vi "RydbergExpControl_2014.09.11_beta.vi"() -> ()   [LabVIEW 2013]
uses:
  AndorCamera/camera_controls.ctl
  <userlib>/atmcd32d.llb/AcquisitionMode_mode typedef.ctl
  <userlib>/atmcd32d.llb/TriggerMode_mode typedef.ctl
  6704/6704_static_voltages_control.ctl
  rydberg_state_machine_states.ctl
panel:
  out "Waveform Chart":dbl(graph)
  in  "Count Number?":bool
  out "Number":dbl format="%^#_6g"
  out "OD":dbl[][](graph)
  out "Atom Closeup":dbl[][](graph)
  out "Atoms - BG":dbl[][](graph)
  out "error out":errorcluster
  out "error constant":errorcluster
  out "Array":dbl[](array[numeric])
  out "Background Image":i16[][](graph)
  out "Atom Image":i16[][](graph)
  in  "Tab Control":T1(tab)
  in  "Trigger Snap Mode":bool
  out "Camera Ready":bool
  in  "Scan Name":string
  in  "Raw_Data Folder":path
  out "Exp Running":bool
  in  "PB Instruction Time To Change":i32
  in  "Static Channel To Change":i32
  in  "Step Size":dbl min=1e-06
  in  "Final Value":dbl
  in  "Initial Value":dbl
  out "You Are Changing:":string
  in  "Shutdown Experiment":bool
  in  "Start Experiment":bool
  in  "Instructions":T2(array[cluster])=[{"Instruct Data"=0, "Op Code"=0, "Flags"=[TRUE, FALSE, FALSE, FALSE, FALSE, FALSE, FALSE, FALSE, FALSE, FALSE, FALSE, FALSE, FALSE, FALSE, FALSE, FALSE, FALSE, FALSE, FALSE, FALSE, FALSE, FALSE, FALSE, FALSE], "Comments"="", "Time (s)"=0.1}, {"Instruct Data"=0, "Op Code"=0, "Flags"=[FALSE, FALSE, FALSE, FALSE, FALSE, FALSE, FALSE, FALSE, FALSE, FALSE, FALSE, FALSE, FALSE, FALSE, FALSE, FALSE, FALSE, FALSE, FALSE, FALSE, FALSE, FALSE, FALSE, FALSE], "Comments"="", "Time (s)"=0.1}, {"Instruct Data"=0, "Op Code"=0, "Flags"=[TRUE, FALSE, FALSE, FALSE, FALSE, FALSE, FALSE, FALSE, FALSE, FALSE, FALSE, FALSE, FALSE, FALSE, FALSE, FALSE, FALSE, FALSE, FALSE, FALSE, FALSE, FALSE, FALSE, FALSE], "Comments"="", "Time (s)"=0.1}, {"Instruct Data"=0, "Op Code"=6, "Flags"=[FALSE, FALSE, FALSE, FALSE, FALSE, FALSE, FALSE, FALSE, FALSE, FALSE, FALSE, FALSE, FALSE, FALSE, FALSE, FALSE, FALSE, FALSE, FALSE, FALSE, FALSE, FALSE, FALSE, FALSE], "Comments"="", "Time (s)"=0.1}] {"Time (s)" format="%.3p"; "Op Code" items=["Continue", "Stop", "Loop", "End Loop", "JSR", "RTS", "Branch", "Long Delay", "Wait"]}
  in  "What To Change":enum16{"PulseBlaster", "Static Voltage"}(ring)=enum."Static Voltage"
  out "Scan Progress":dbl(slide) caption="Slide" scale=0.0..100.0
  out "Camera Information":T3 {"VS Speed (us)" format="%.2f"}
  in  "Acquisition Parameters":T4={"Acquisition Mode"=enum."Kinetics", "Trigger Mode"=enum."External", "Frame \nTransfer"=FALSE, "Exposure Time (s)"=0.0001, "Accumulation Cycle Time (s)"=0.0, "# Accumulations"=1, "# Kinetics"=2, "Kinetic Cycle Time (s)"=0.0, "Horizontal Bin Size"=1, "Vertical Bin Size"=1} {"Vertical Bin Size" min=1; "Horizontal Bin Size" min=1; "Kinetic Cycle Time (s)" format="%.2f"; "# Kinetics" min=1; "# Accumulations" min=1; "Accumulation Cycle Time (s)" format="%.2f"; "Exposure Time (s)" format="%.2e"}
  out "Calcualted Times":T7 {"Kinetic" format="%.4f"; "Accumulate" format="%.4f"; "Exposure" format="%.4f"}
  in  "Red MOT 87 Inputs":T8={"Active Device"="6733_Red_87", "Active Channels"=[TRUE, FALSE, FALSE, FALSE, FALSE, FALSE, FALSE, FALSE], "Waveform Parameters"=[[{"Functional Form"=enum."Polynomial", "Start Voltage"=0.0, "End Voltage"=0.0, "Time"=0.0, "Degree"=1, "Sample Rate"=0.0}, {"Functional Form"=enum."Exponential", "Start Voltage"=0.0, "End Voltage"=0.0, "Time"=0.0, "Degree"=1, "Sample Rate"=0.0}, {"Functional Form"=enum."Exponential", "Start Voltage"=0.0, "End Voltage"=0.0, "Time"=0.0, "Degree"=1, "Sample Rate"=0.0}, {"Functional Form"=enum."Exponential", "Start Voltage"=0.0, "End Voltage"=0.0, "Time"=0.0, "Degree"=1, "Sample Rate"=0.0}, {"Functional Form"=enum."Exponential", "Start Voltage"=0.0, "End Voltage"=0.0, "Time"=0.0, "Degree"=1, "Sample Rate"=0.0}, {"Functional Form"=enum."Exponential", "Start Voltage"=0.0, "End Voltage"=0.0, "Time"=0.0, "Degree"=1, "Sample Rate"=0.0}], [{"Functional Form"=enum."Exponential", "Start Voltage"=0.0, "End Voltage"=0.0, "Time"=0.0, "Degree"=1, "Sample Rate"=0.0}, {"Functional Form"=enum."Exponential", "Start Voltage"=0.0, "End Voltage"=0.0, "Time"=0.0, "Degree"=1, "Sample Rate"=0.0}, {"Functional Form"=enum."Exponential", "Start Voltage"=0.0, "End Voltage"=0.0, "Time"=0.0, "Degree"=1, "Sample Rate"=0.0}, {"Functional Form"=enum."Exponential", "Start Voltage"=0.0, "End Voltage"=0.0, "Time"=0.0, "Degree"=1, "Sample Rate"=0.0}, {"Functional Form"=enum."Exponential", "Start Voltage"=0.0, "End Voltage"=0.0, "Time"=0.0, "Degree"=1, "Sample Rate"=0.0}, {"Functional Form"=enum."Exponential", "Start Voltage"=0.0, "End Voltage"=0.0, "Time"=0.0, "Degree"=1, "Sample Rate"=0.0}], [{"Functional Form"=enum."Exponential", "Start Voltage"=0.0, "End Voltage"=0.0, "Time"=0.0, "Degree"=1, "Sample Rate"=0.0}, {"Functional Form"=enum."Exponential", "Start Voltage"=0.0, "End Voltage"=0.0, "Time"=0.0, "Degree"=1, "Sample Rate"=0.0}, {"Functional Form"=enum."Exponential", "Start Voltage"=0.0, "End Voltage"=0.0, "Time"=0.0, "Degree"=1, "Sample Rate"=0.0}, {"Functional Form"=enum."Exponential", "Start Voltage"=0.0, "End Voltage"=0.0, "Time"=0.0, "Degree"=1, "Sample Rate"=0.0}, {"Functional Form"=enum."Exponential", "Start Voltage"=0.0, "End Voltage"=0.0, "Time"=0.0, "Degree"=1, "Sample Rate"=0.0}, {"Functional Form"=enum."Exponential", "Start Voltage"=0.0, "End Voltage"=0.0, "Time"=0.0, "Degree"=1, "Sample Rate"=0.0}], [{"Functional Form"=enum."Exponential", "Start Voltage"=0.0, "End Voltage"=0.0, "Time"=0.0, "Degree"=1, "Sample Rate"=0.0}, {"Functional Form"=enum."Exponential", "Start Voltage"=0.0, "End Voltage"=0.0, "Time"=0.0, "Degree"=1, "Sample Rate"=0.0}, {"Functional Form"=enum."Exponential", "Start Voltage"=0.0, "End Voltage"=0.0, "Time"=0.0, "Degree"=1, "Sample Rate"=0.0}, {"Functional Form"=enum."Exponential", "Start Voltage"=0.0, "End Voltage"=0.0, "Time"=0.0, "Degree"=1, "Sample Rate"=0.0}, {"Functional Form"=enum."Exponential", "Start Voltage"=0.0, "End Voltage"=0.0, "Time"=0.0, "Degree"=1, "Sample Rate"=0.0}, {"Functional Form"=enum."Exponential", "Start Voltage"=0.0, "End Voltage"=0.0, "Time"=0.0, "Degree"=1, "Sample Rate"=0.0}], [{"Functional Form"=enum."Exponential", "Start Voltage"=0.0, "End Voltage"=0.0, "Time"=0.0, "Degree"=1, "Sample Rate"=0.0}, {"Functional Form"=enum."Exponential", "Start Voltage"=0.0, "End Voltage"=0.0, "Time"=0.0, "Degree"=1, "Sample Rate"=0.0}, {"Functional Form"=enum."Exponential", "Start Voltage"=0.0, "End Voltage"=0.0, "Time"=0.0, "Degree"=1, "Sample Rate"=0.0}, {"Functional Form"=enum."Exponential", "Start Voltage"=0.0, "End Voltage"=0.0, "Time"=0.0, "Degree"=1, "Sample Rate"=0.0}, {"Functional Form"=enum."Exponential", "Start Voltage"=0.0, "End Voltage"=0.0, "Time"=0.0, "Degree"=1, "Sample Rate"=0.0}, {"Functional Form"=enum."Exponential", "Start Voltage"=0.0, "End Voltage"=0.0, "Time"=0.0, "Degree"=1, "Sample Rate"=0.0}], [{"Functional Form"=enum."Exponential", "Start Voltage"=0.0, "End Voltage"=0.0, "Time"=0.0, "Degree"=1, "Sample Rate"=0.0}, {"Functional Form"=enum."Exponential", "Start Voltage"=0.0, "End Voltage"=0.0, "Time"=0.0, "Degree"=1, "Sample Rate"=0.0}, {"Functional Form"=enum."Exponential", "Start Voltage"=0.0, "End Voltage"=0.0, "Time"=0.0, "Degree"=1, "Sample Rate"=0.0}, {"Functional Form"=enum."Exponential", "Start Voltage"=0.0, "End Voltage"=0.0, "Time"=0.0, "Degree"=1, "Sample Rate"=0.0}, {"Functional Form"=enum."Exponential", "Start Voltage"=0.0, "End Voltage"=0.0, "Time"=0.0, "Degree"=1, "Sample Rate"=0.0}, {"Functional Form"=enum."Exponential", "Start Voltage"=0.0, "End Voltage"=0.0, "Time"=0.0, "Degree"=1, "Sample Rate"=0.0}], [{"Functional Form"=enum."Exponential", "Start Voltage"=0.0, "End Voltage"=0.0, "Time"=0.0, "Degree"=1, "Sample Rate"=0.0}, {"Functional Form"=enum."Exponential", "Start Voltage"=0.0, "End Voltage"=0.0, "Time"=0.0, "Degree"=1, "Sample Rate"=0.0}, {"Functional Form"=enum."Exponential", "Start Voltage"=0.0, "End Voltage"=0.0, "Time"=0.0, "Degree"=1, "Sample Rate"=0.0}, {"Functional Form"=enum."Exponential", "Start Voltage"=0.0, "End Voltage"=0.0, "Time"=0.0, "Degree"=1, "Sample Rate"=0.0}, {"Functional Form"=enum."Exponential", "Start Voltage"=0.0, "End Voltage"=0.0, "Time"=0.0, "Degree"=1, "Sample Rate"=0.0}, {"Functional Form"=enum."Exponential", "Start Voltage"=0.0, "End Voltage"=0.0, "Time"=0.0, "Degree"=1, "Sample Rate"=0.0}], [{"Functional Form"=enum."Exponential", "Start Voltage"=0.0, "End Voltage"=0.0, "Time"=0.0, "Degree"=1, "Sample Rate"=0.0}, {"Functional Form"=enum."Exponential", "Start Voltage"=0.0, "End Voltage"=0.0, "Time"=0.0, "Degree"=1, "Sample Rate"=0.0}, {"Functional Form"=enum."Exponential", "Start Voltage"=0.0, "End Voltage"=0.0, "Time"=0.0, "Degree"=1, "Sample Rate"=0.0}, {"Functional Form"=enum."Exponential", "Start Voltage"=0.0, "End Voltage"=0.0, "Time"=0.0, "Degree"=1, "Sample Rate"=0.0}, {"Functional Form"=enum."Exponential", "Start Voltage"=0.0, "End Voltage"=0.0, "Time"=0.0, "Degree"=1, "Sample Rate"=0.0}, {"Functional Form"=enum."Exponential", "Start Voltage"=0.0, "End Voltage"=0.0, "Time"=0.0, "Degree"=1, "Sample Rate"=1.0}]], "Active Phases"=[TRUE, FALSE, FALSE, FALSE, FALSE, FALSE], "Phase Times"=[0.001], "Trigger Channel"="/6733_Red_87/PFI0"} {"Phase Times" format="%.0p"; "Waveform Parameters"."Degree" min=1}
  in  "6704 Static Voltage Settings":T9={"Device Name"="6704_Static", "Voltages"=[5.0, 0.0, 0.0, 0.0, 0.0, 0.0, 0.0, 0.0, 0.0, 0.0, 0.0, 0.0, 0.0, 0.0, 0.0, 0.0]}
  out "Andor Initialization Error Codes":T10
  out "Acq. Error Codes":T11
  out "Tree":string(tree)
  # "(1) 461 MOT beams"
  # "(2) Imaging AOM 1"
  # "(3) Imaging AOM 2"
  # "(4) Camera"
  # "(5) Zeeman shutter"
  # "(6) Repumper shutter"
  # "(7) 461 MOT coils"
  # "(8) 689 MOT coils"
  # "(9) 87 Sr Red MOT Trig"
  # "(10) ??? Shutter"
  # "(11) Red AOM"
  # "(12) Sat Abs Current Switch"
  # "(13) Zeeman MOSFET"
  # "1"
  # "2"
  # "3"
  # "4"
  # "5"
  # "6"
  # "7"
  # "8"
  # "9"
  # "10"
  # "11"
  # "12"
  # "13"
  # "14"
  # "15"
  # "16"
  # "17"
  # "18"
  # "19"
  # "20"
  # "21"
  # "22"
  # "23"
  # "24"
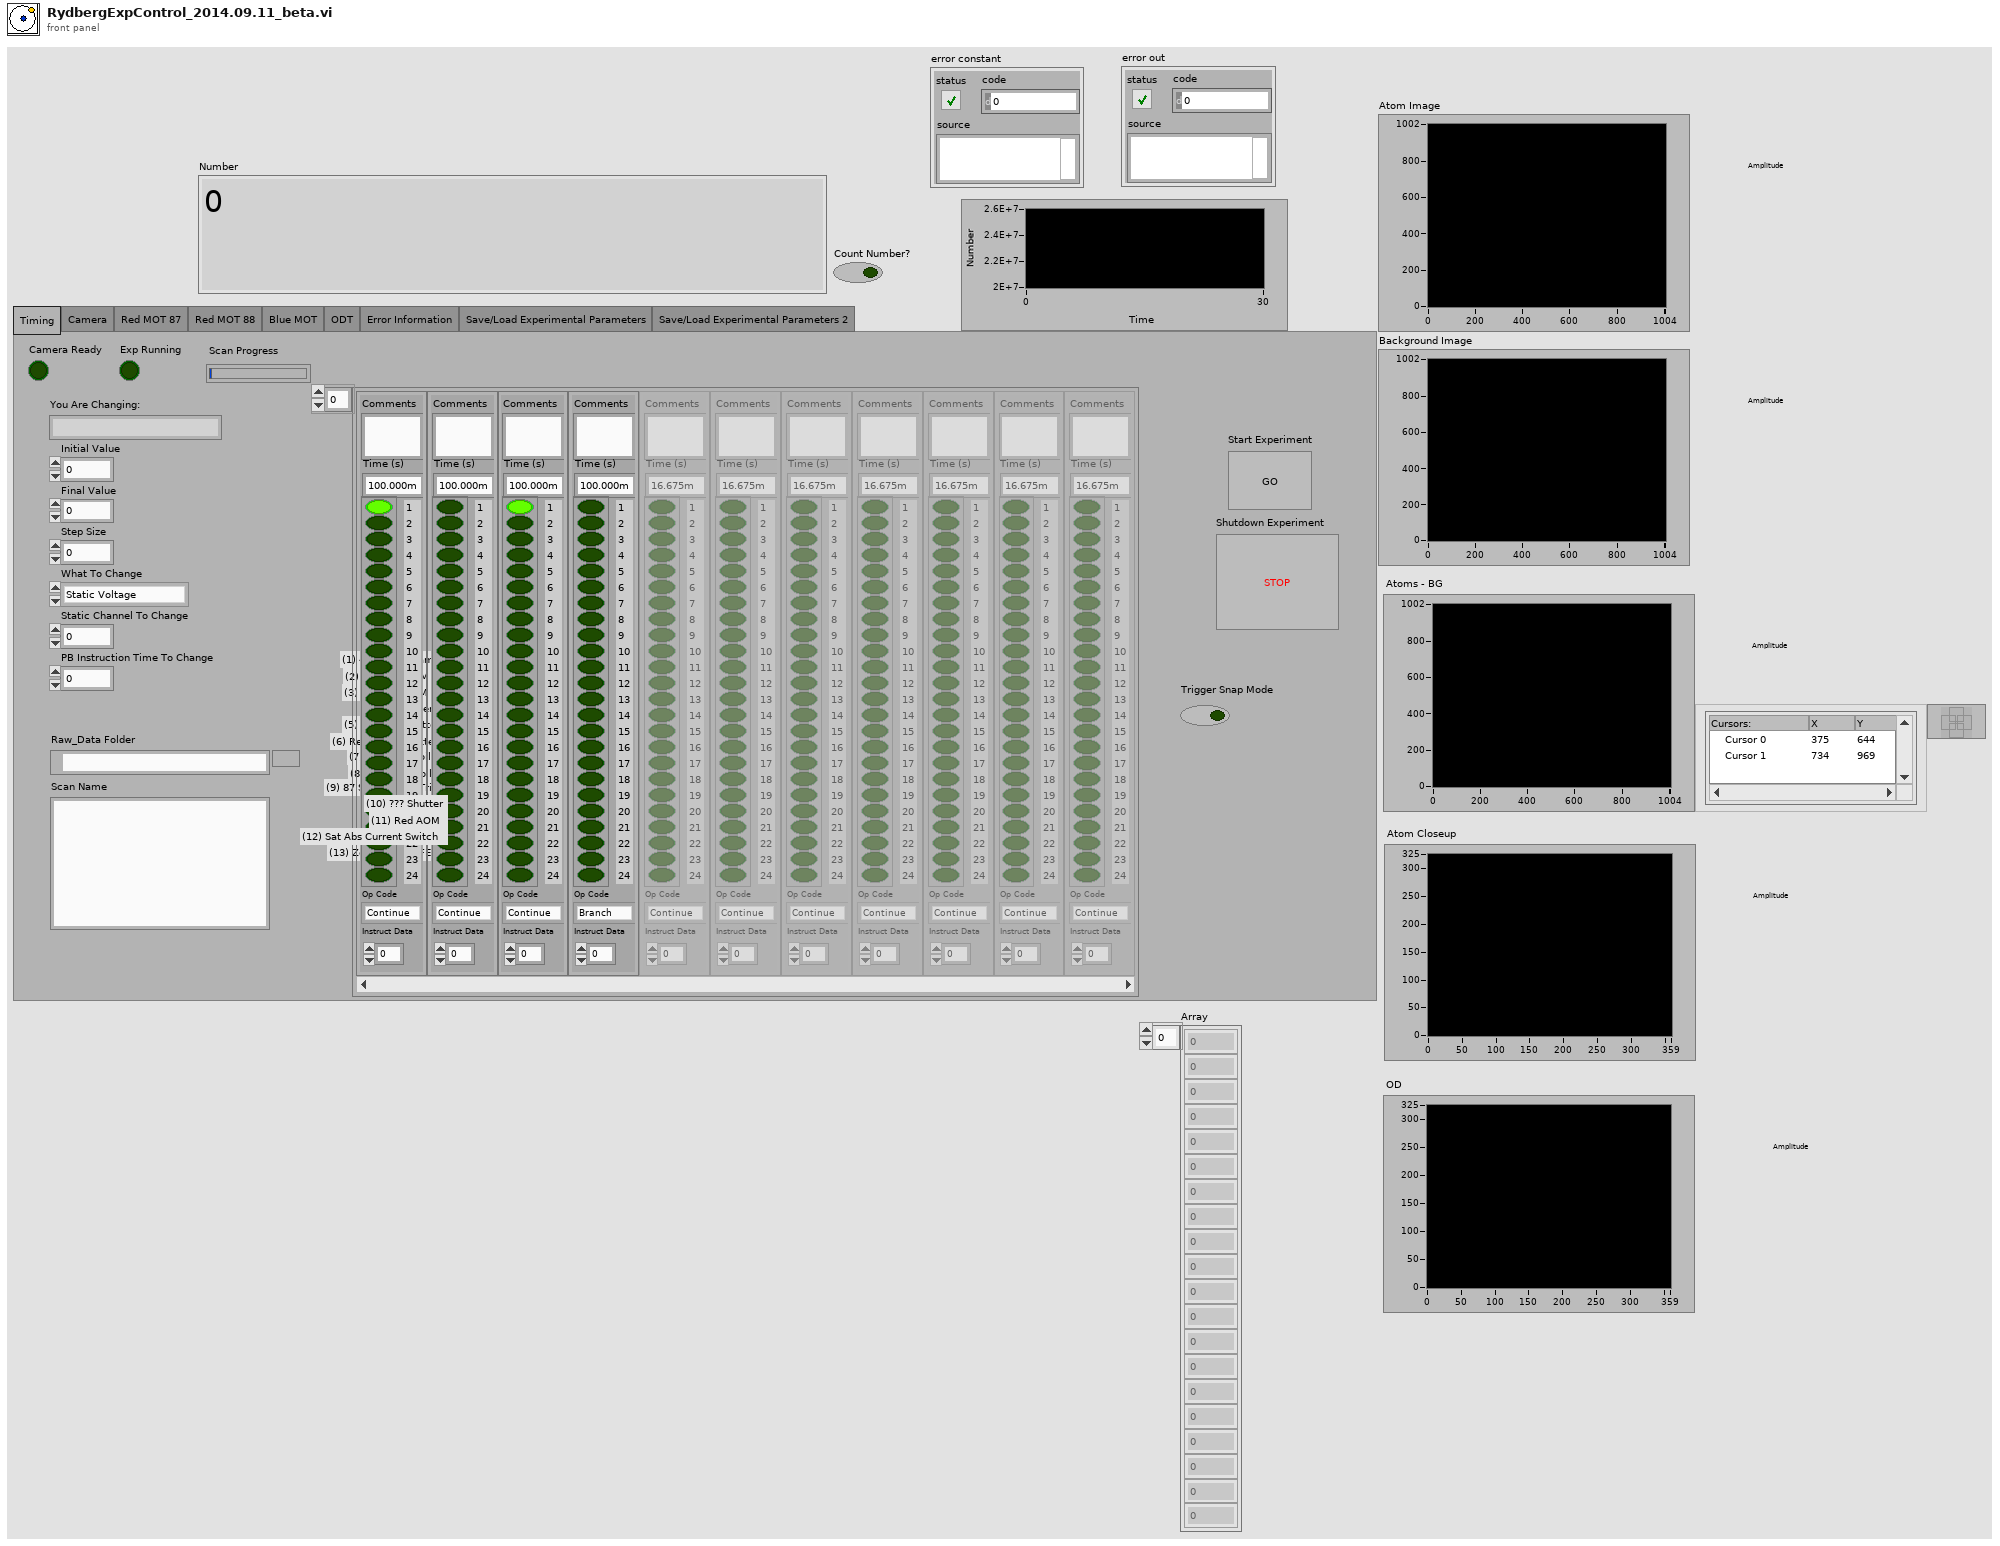
[diagram p1: front panel]
types:
  T1 = enum32{"Timing", "Camera", "Red MOT 87", "Red MOT 88", "Blue MOT", "ODT", "Error Information", "Save/Load Experimental Parameters", "Save/Load Experimental Parameters 2"}
  T2 = cluster{"Instruct Data":i32, "Op Code":i32, "Flags":bool[], "Comments":string, "Time (s)":dbl}[]
  T3 = cluster{"xpixels":i32, "ypixels":i32, "# VS Speeds":i32, "VS Speed (us)":sgl, "Temperature Stable":bool, "Temperature (C)":i32}
  T4 = typedef "camera_controls.ctl" = cluster{"Acquisition Mode":T5, "Trigger Mode":T6, "Frame \nTransfer":bool, "Exposure Time (s)":sgl, "Accumulation Cycle Time (s)":sgl, "# Accumulations":i32, "# Kinetics":i32, "Kinetic Cycle Time (s)":sgl, "Horizontal Bin Size":i32, "Vertical Bin Size":i32}
  T5 = typedef "AcquisitionMode_mode typedef.ctl" = enum16{"Reserved (0)", "Single Scan", "Accumulate", "Kinetics", "Fast Kinetics", "Run Till Abort", "Reserved (6)", "Reserved (7)", "Reserved (8)", "Time Delayed Integration"}
  T6 = typedef "TriggerMode_mode typedef.ctl" = enum16{"Internal", "External", "N/A (2)", "N/A (3)", "N/A (4)", "N/A (5)", "External Start", "External Exposure (Bulb)", "N/A (8)", "External FVB EM", "Software", "N/A (11)", "External Charge Shifting"}
  T7 = cluster{"Exposure":sgl, "Accumulate":sgl, "Kinetic":sgl}
  T8 = cluster{"Active Device":string, "Active Channels":bool[], "Waveform Parameters":cluster{"Functional Form":enum16{"Polynomial", "Exponential"}, "Start Voltage":dbl, "End Voltage":dbl, "Time":dbl, "Degree":i8, "Sample Rate":dbl}[][], "Active Phases":bool[], "Phase Times":dbl[], "Trigger Channel":tag}
  T9 = typedef "6704_static_voltages_control.ctl" = cluster{"Device Name":string, "Voltages":dbl[]}
  T10 = cluster{"Initalize Error Code":u32, "GetDetector Error Code":u32, "Get#VSSpeeds Error Code":u32, "Set VS Speed Error":u32, "CoolerOn Error Code":u32, "GetTemperature Error Code":u32, "Shutdown Error Code":u32}
  T11 = cluster{"Set Acq. Mode Error":u32, "Set Trigger Mode Error":u32, "Set FT Error Code":u32, "Set Exposure Time Error Code":u32, "Set Accum Time Error":u32, "Set # Accum Error":u32, "Set # Kinetics Error":u32, "SetKinCycleTime Error":u32}
  T12 = typedef "rydberg_state_machine_states.ctl" = enum16{"Initialize", "Idle", "Trigger Snap Mode", "Scan Mode", "Load Experiment", "Shutdown"}
  T13 = cluster{"6704 Static Voltage Settings":T9, "Instructions":cluster{"Instruct Data":i32, "Op Code":i32, "Flags":bool[], "Comments":string, "Time (s)":dbl}[], "Red MOT 87 Inputs":cluster{"Active Device":string, "Active Channels":bool[], "Waveform Parameters":cluster{"Functional Form":enum16{"Polynomial", "Exponential"}, "Start Voltage":dbl, "End Voltage":dbl, "Time":dbl, "Degree":i8, "Sample Rate":dbl}[][], "Active Phases":bool[], "Phase Times":dbl[], "Trigger Channel":tag}}
  T14 = typedef "LVCursorListTypeDef.ctl" = cluster{"Name":string, "Color":u32, "Style":u8, "Point Style":u8, "Name Visible":bool, "Allow Drag":bool, "Cursor Mode":u32, "Plot":i32, "Index":i32, "Position":cluster{"X":dbl, "Y":dbl}, "X Scale":u32, "Y Scale":u32, "Watch Plots":i32[], "Watch All Plots":bool, "Plot Area":i32, "Label Offset":cluster{"X":dbl, "Y":dbl}}[]
  T15 = cluster{"Instruct Data":i32, "Op Code":i32, "Flags":bool[], "Comments":string, "Time (s)":dbl}
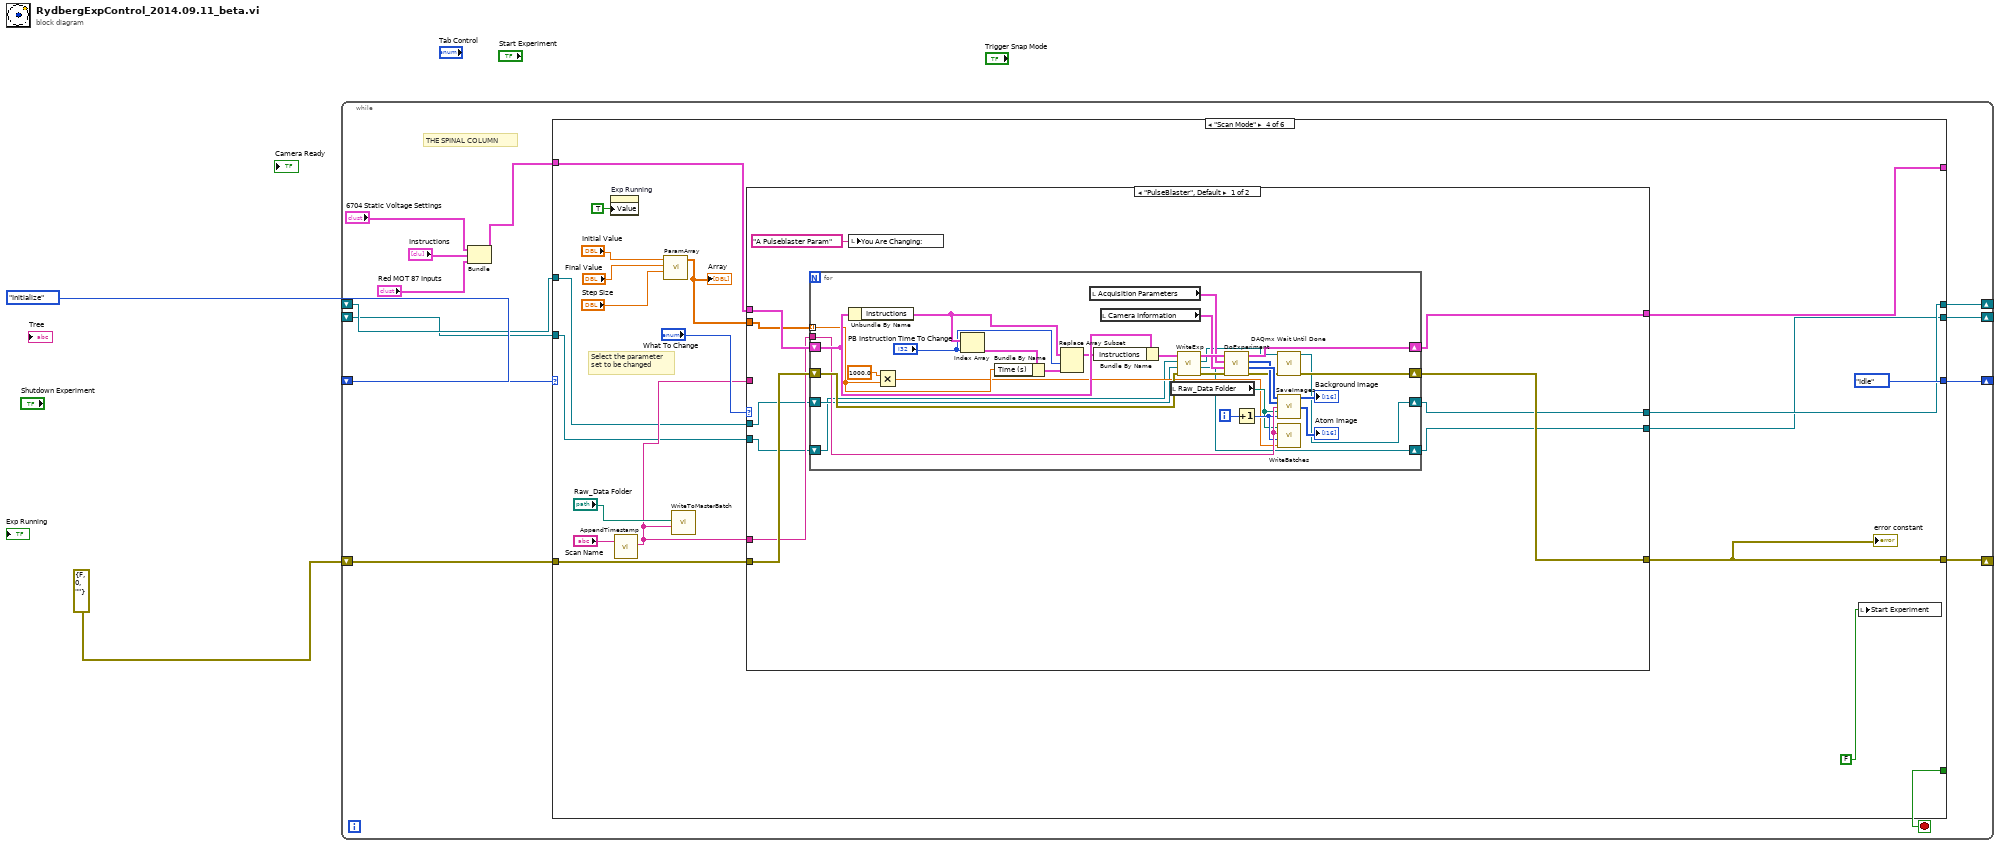
[diagram p0: block diagram]
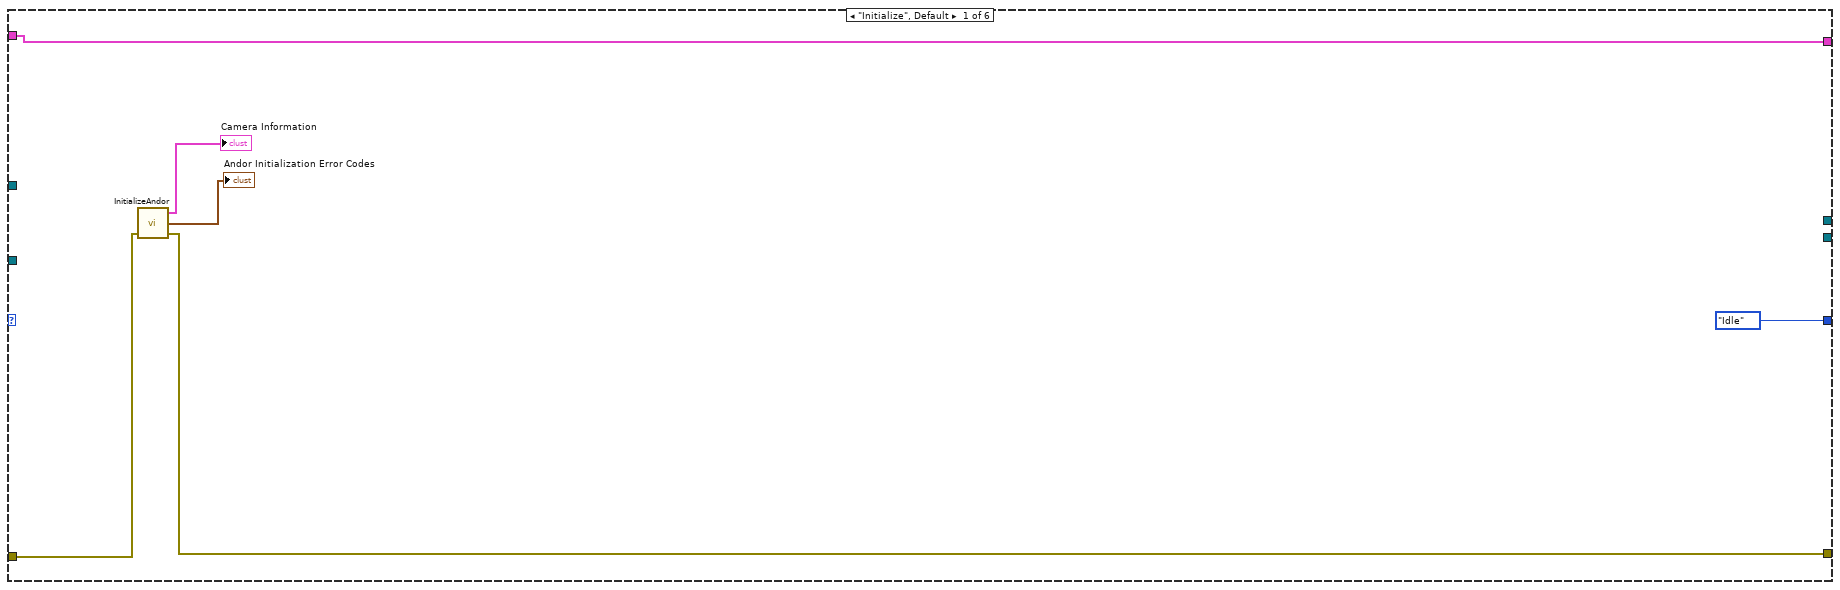
[diagram p2: hidden frame]
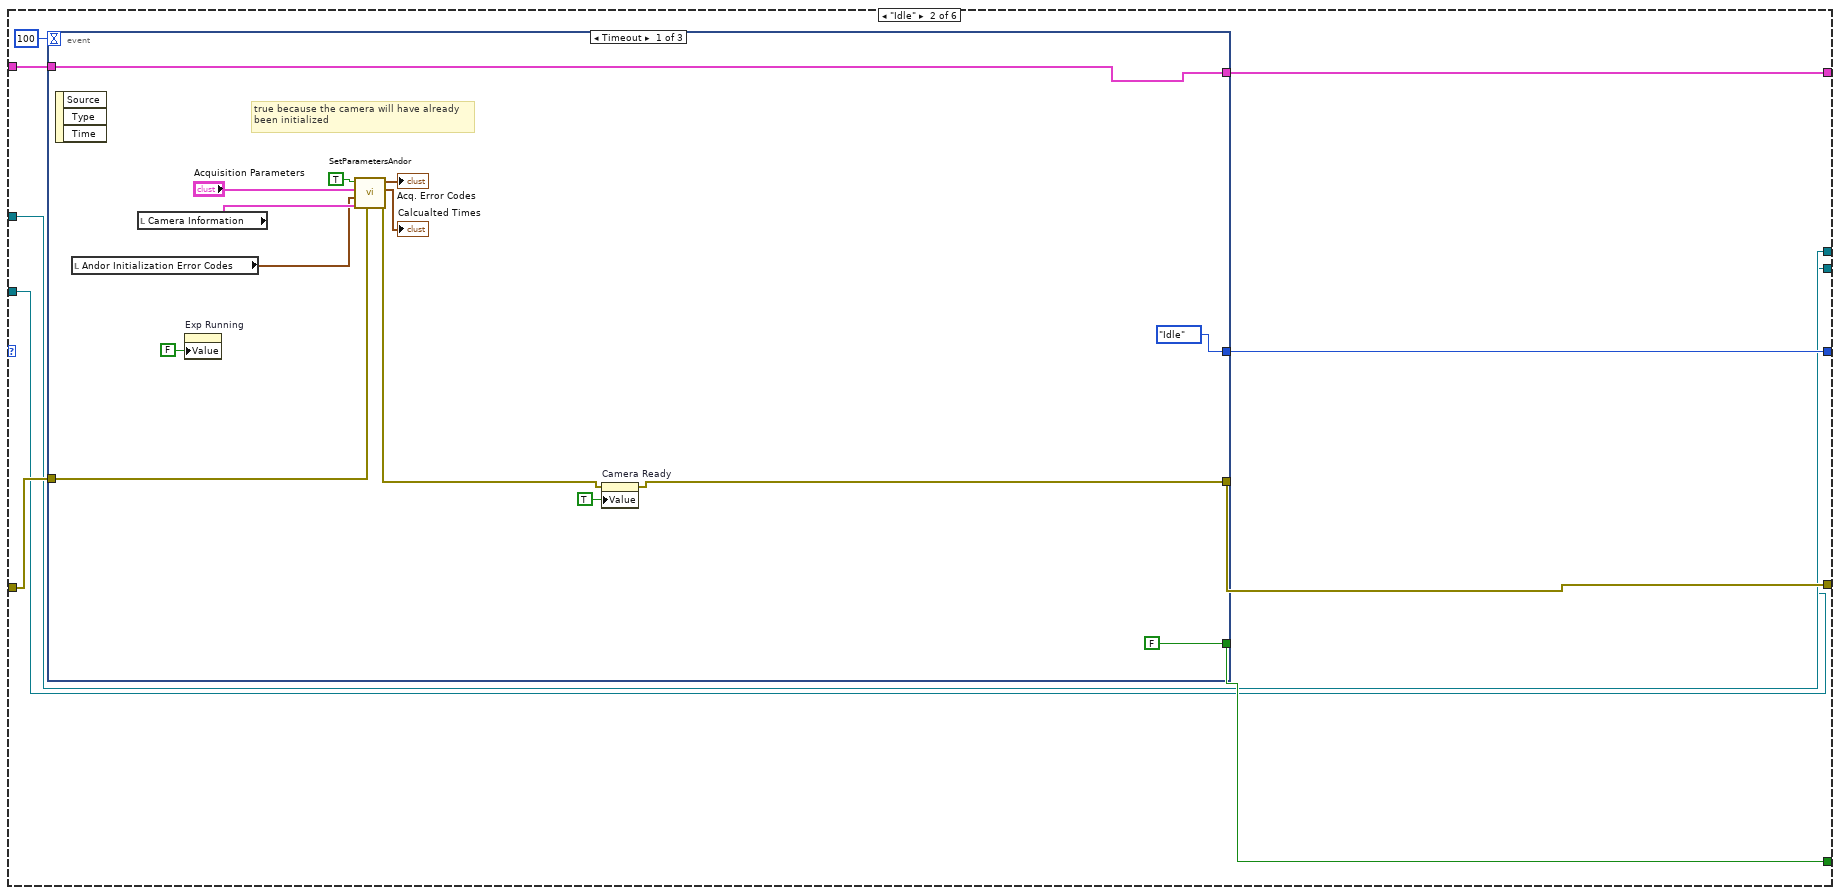
[diagram p3: hidden frame]
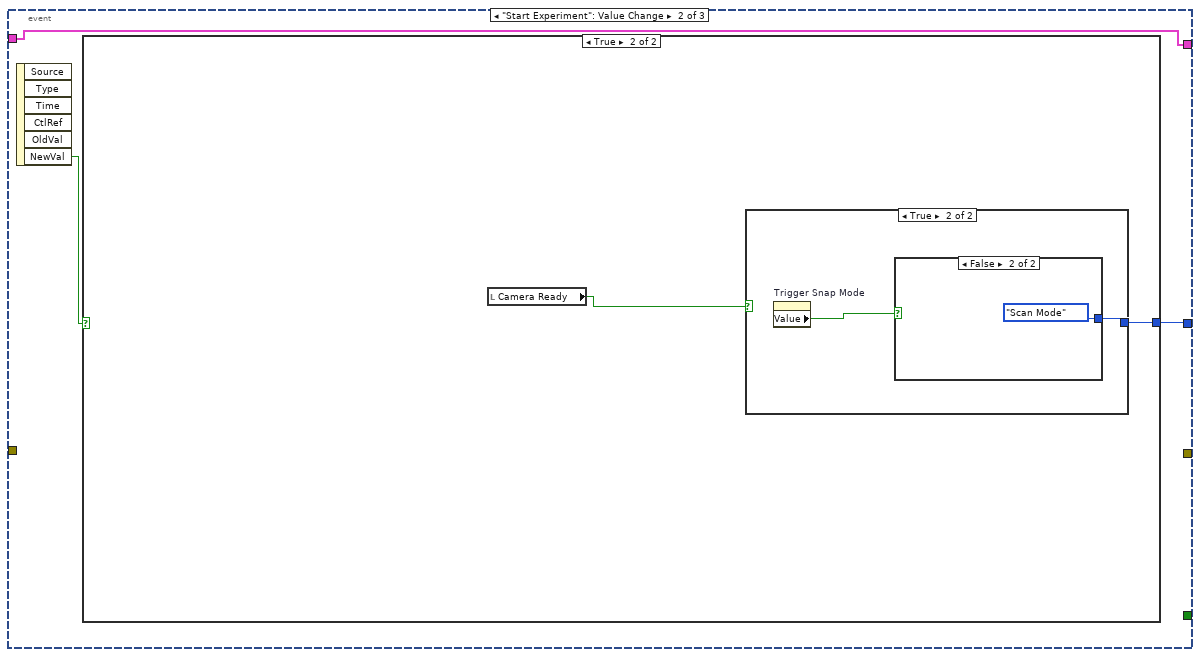
[diagram p4: hidden frame]
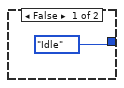
[diagram p5: hidden frame]
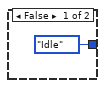
[diagram p6: hidden frame]
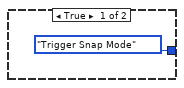
[diagram p7: hidden frame]
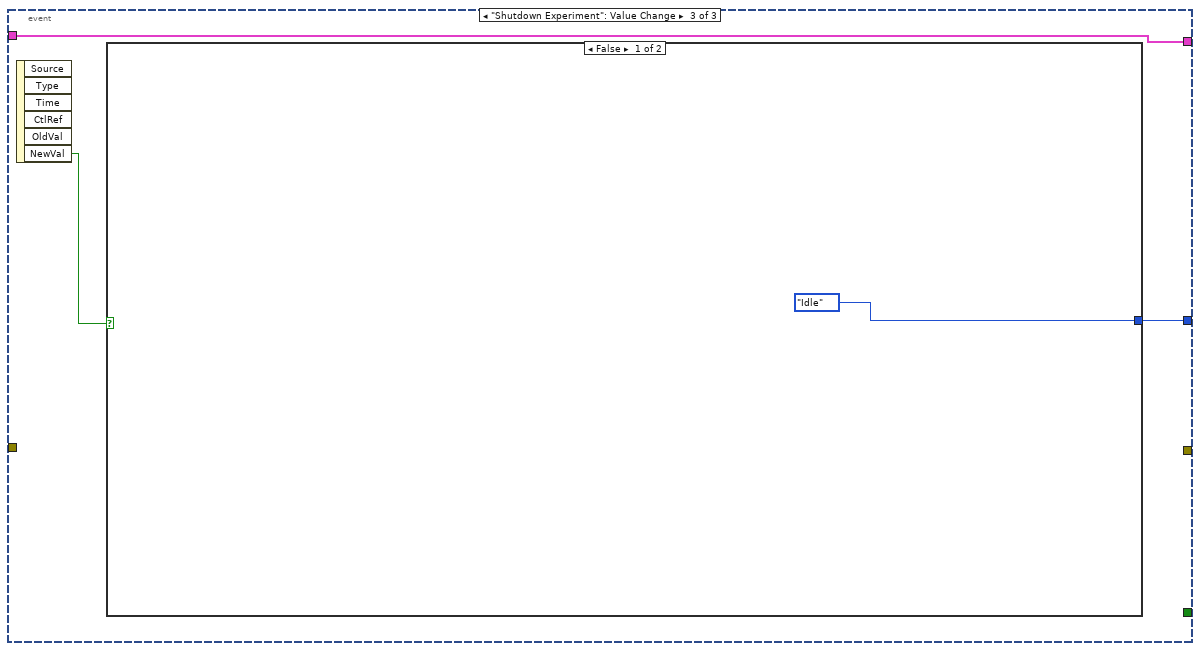
[diagram p8: hidden frame]
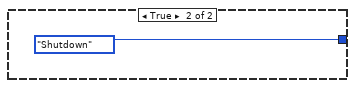
[diagram p9: hidden frame]
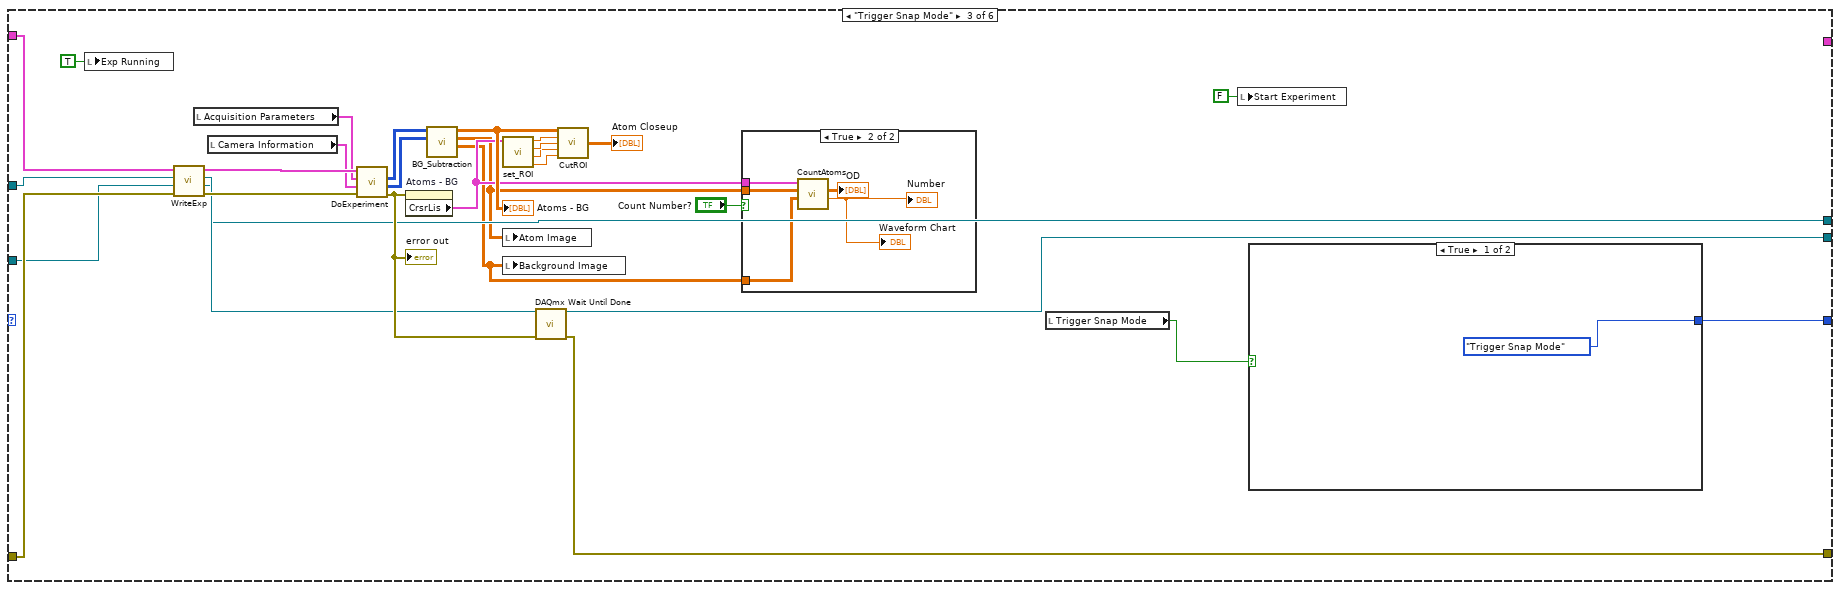
[diagram p10: hidden frame]
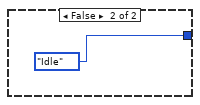
[diagram p12: hidden frame]
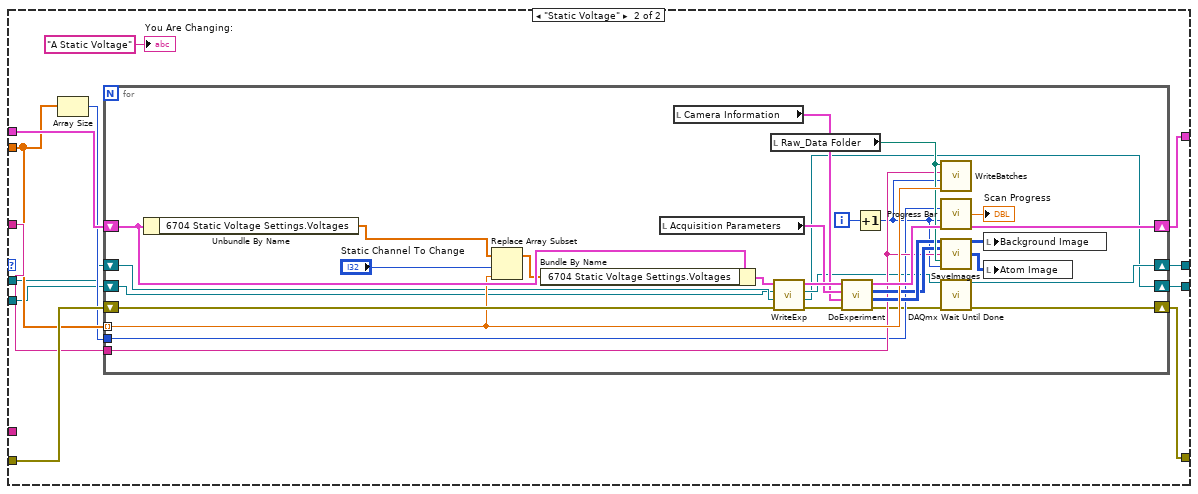
[diagram p13: hidden frame]
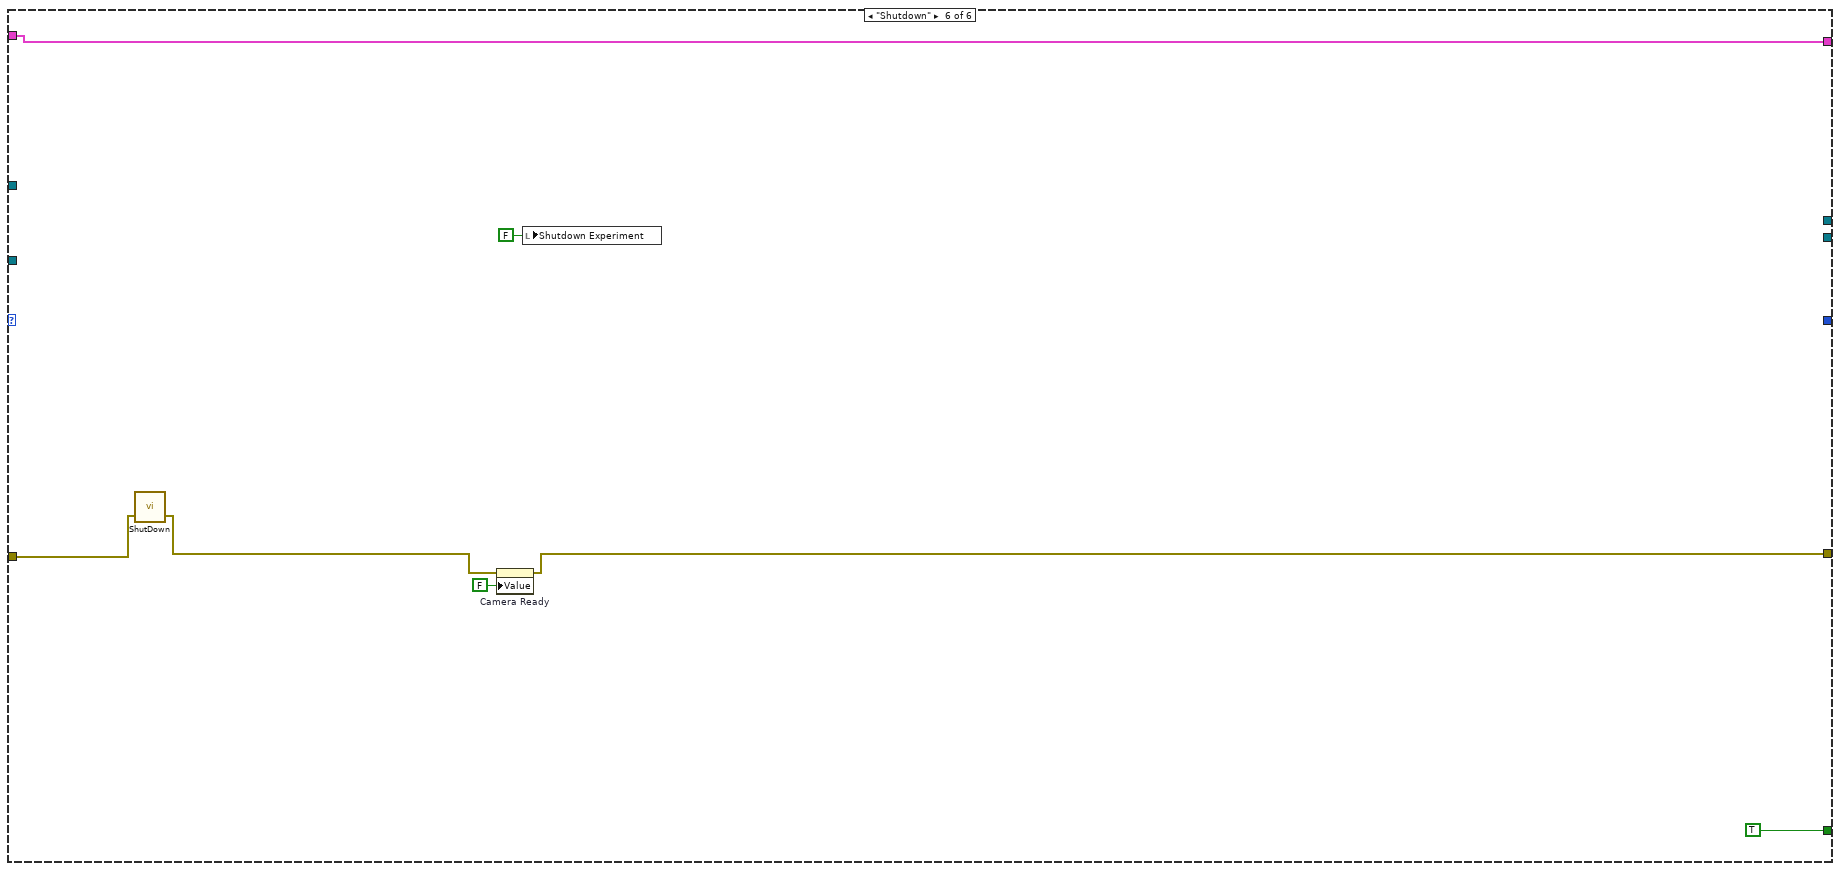
[diagram p15: hidden frame]
diagram:
  n1 = while {
    shift-right: [w12] -> _
    shift-left: rydberg_state_machine_states."Initialize" -> [w15]
    shift-right: [w13] -> _
    shift-left: errorcluster {"status"=FALSE, "code"=0, "source"=""} ("error constant") -> [w14]
    shift-right: [w6] -> _
    shift-left: _ -> [w5]
    shift-right: [w4] -> _
    shift-left: _ -> [w3]
    stop <- w11 stop-if-true
    # "THE SPINAL COLUMN"
    n2 = Bundle("6704 Static Voltage Settings"="6704 Static Voltage Settings", "Instructions"="Instructions", "Red MOT 87 Inputs"="Red MOT 87 Inputs") -> (w7:T13)  [unwired: 1 in]
    n3 = case shown="\"Scan Mode\"" w15 {
      tunnel: w14 -> [w21 w30 w89 w107 _ w206]
      tunnel: [w18 w26 w65 w106 _ w201] -> w13
      tunnel: [rydberg_state_machine_states."Idle" w28 w75 rydberg_state_machine_states."Idle" _ _] -> w12
      tunnel: [_ w27 _ _ _ TRUE] -> w11
      tunnel: [w16 w25 _ w109 w199 w203] -> _
      tunnel: w7 -> [w16 w24 w88 w110 w199 w203]
      tunnel: [_ w23 w69 w98 _ _] -> w6
      tunnel: w5 -> [_ w23 w68 w100 _ _]
      tunnel: [_ w22 w67 w97 _ _] -> w4
      tunnel: w3 -> [_ w22 w66 w99 _ _]
      frame "Initialize", Default {
        n4 = call "InitializeAndor.vi"("Error In"=w21) -> ("error out"=w18:errorcluster, "Andor Initialization Error Codes"=→"Andor Initialization Error Codes":T10, "Camera Information"=→"Camera Information":T3)  [unwired: 2 in]
      }
      frame "Idle" {
        n5 = event shown="[0] Timeout" {
          selector: _ -> [_ _ _]
          dyn-events: _ -> [_ _ _]
          timeout: 100 -> [_ _ _]
          tunnel: w30 -> [w38 _ _]
          tunnel: [rydberg_state_machine_states."Idle" w46 w57] -> w28
          tunnel: [FALSE _ _] -> w27
          tunnel: [w32 _ _] -> w26
          tunnel: [w35 w45 w56] -> w25
          tunnel: w24 -> [w35 w45 w56]
          event Timeout {
            # "true because the camera will have already\nbeen initialized"
            n6 = event-data() -> ()  [unwired: 1 in, 3 out]
            n7 = local read "Andor Initialization Error Codes"() -> (w37:T10)
            n8 = local read "Camera Information"() -> (w40:T3)
            n9 = property on="Exp Running" class="Bool (strict)"("Value"=FALSE ("Exp Running")) -> ()  [unwired: 2 in, 2 out]
            n10 = call "SetParametersAndor.vi"("Error In"=w38, "Camera Information"=w40, "Andor Initialization Error Codes"=w37, "Acquisition Parameters"="Acquisition Parameters", "Pre Initialized?"=TRUE) -> ("error out"=w33:errorcluster, "Calcualted Times"=→"Calcualted Times":T7, "Acq. Error Codes"=→"Acq. Error Codes":T11)  [unwired: 4 in]
            n11 = property on="Camera Ready" class="Bool (strict)"(error in=w33, "Value"=TRUE ("Camera Ready")) -> (error out=w32:errorcluster)  [unwired: 1 in, 1 out]
          }
          event "Start Experiment": Value Change {
            n12 = event-data() -> ("NewVal"=w47:bool)  [unwired: 1 in, 5 out]
            n13 = case shown="True" w47 {
              tunnel: [rydberg_state_machine_states."Idle" w50] -> w46
              frame False {
              }
              frame True {
                n14 = local read "Camera Ready"() -> (w49:bool)
                n15 = case shown="True" w49 {
                  tunnel: [rydberg_state_machine_states."Idle" w53] -> w50
                  frame False {
                  }
                  frame True {
                    n16 = property on="Trigger Snap Mode" class="Bool (strict)"() -> ("Value"=w52:bool)  [unwired: 2 in, 2 out]
                    n17 = case shown="False" w52 {
                      tunnel: [rydberg_state_machine_states."Trigger Snap Mode" rydberg_state_machine_states."Scan Mode"] -> w53
                      frame True {
                      }
                      frame False {
                      }
                    }
                  }
                }
              }
            }
          }
          event "Shutdown Experiment": Value Change {
            n18 = event-data() -> ("NewVal"=w58:bool)  [unwired: 1 in, 5 out]
            n19 = case shown="False" w58 {
              tunnel: [rydberg_state_machine_states."Idle" rydberg_state_machine_states."Shutdown"] -> w57
              frame False {
              }
              frame True {
              }
            }
          }
        }
      }
      frame "Trigger Snap Mode" {
        n20 = local write "Exp Running"(TRUE ("Exp Running")) -> ()
        n21 = call "WriteExp.vi"("error in (no error)"=w89, "Control Task In"=w66, "Waveform Task In"=w68, "Experimental Control Cluster In"=w88) -> ("error out"=w72:errorcluster, "waveform task out"=w69:refnum<k21>, "counter task out"=w70:refnum<k21>, "Experimental Control Cluster Out"=w87:T13)  [unwired: 4 in]
        n22 = local read "Acquisition Parameters"() -> (w86:T4)
        n23 = local read "Camera Information"() -> (w85:T3)
        n24 = call "DoExperiment.vi"("Error In"=w72, "Camera Information 2"=w85, "Acquisition Parameters"=w86, "output cluster"=w87) -> ("error out"=w71:errorcluster, "Background Image"=w83:i32[][], "Atom Image"=w84:i32[][])  [unwired: 4 in, 1 out]
        "error out" <- w71
        n25 = property on="Atoms - BG" class="IntGraph (strict)"(error in=w71) -> ("CrsrLis"=w64:T14)  [unwired: 1 in, 2 out]
        n26 = call "BG_Subtraction.vi"("Background Image"=w83, "Atom Image"=w84) -> ("Background Image Out"=w62:dbl[][], "Atom Image Out"=w63:dbl[][], "Atoms - BG"=w81:dbl[][])  [unwired: 7 in]
        "Atoms - BG" <- w81
        n27 = call "set_ROI.vi"("Cursor List"=w64) -> ("Row End"=w77:dbl, "RowStart"=w78:dbl, "ColEnd"=w79:dbl, "ColStart"=w80:dbl)  [unwired: 7 in]
        n28 = local write "Atom Image"(w63) -> ()
        n29 = local write "Background Image"(w62) -> ()
        n30 = call <vilib>:"DAQmx Wait Until Done.vi"("task/channels in"=w70, "error in"=w71) -> ("task out"=w67:refnum<k21>, "error out"=w65:errorcluster)  [unwired: 12 in]
        n31 = call "CutROI.vi"("Full Image In"=w81, "Col Start"=w80, "Col End"=w79, "Row Start"=w78, "Row End"=w77) -> ("Cut Image Out"=→"Atom Closeup":dbl[][])  [unwired: 10 in]
        n32 = case shown="True" "Count Number?" {
          tunnel: w64 -> [_ w93]
          tunnel: w63 -> [_ w92]
          tunnel: w62 -> [_ w91]
          frame False {
          }
          frame True {
            n33 = call "CountAtoms.vi"("Background Image"=w91, "Atom Image"=w92, "Cursor List"=w93) -> ("Number"=→"Number" →"Waveform Chart":dbl, "OD"=→"OD":dbl[][])  [unwired: 7 in]
          }
        }
        n34 = local read "Trigger Snap Mode"() -> (w76:bool)
        n35 = local write "Start Experiment"(FALSE ("Start Experiment")) -> ()
        n36 = case shown="True" w76 {
          tunnel: [rydberg_state_machine_states."Trigger Snap Mode" rydberg_state_machine_states."Idle"] -> w75
          frame True {
          }
          frame False {
          }
        }
      }
      frame "Scan Mode" {
        # "Select the parameter\nset to be changed"
        n37 = property on="Exp Running" class="Bool (strict)"("Value"=TRUE ("Exp Running")) -> ()  [unwired: 2 in, 2 out]
        n38 = call "AppendTimestamp.vi"("String"="Scan Name") -> ("String 2"=w101:string)  [unwired: 10 in]
        n39 = call "ParamArray.vi"("Step Size"="Step Size", "Final Value"="Final Value", "Initial Value"="Initial Value") -> ("Array"=w108:dbl[])  [unwired: 8 in]
        "Array" <- w108
        n40 = call "WriteToMasterBatch.vi"("Scan name"=w101, "Raw_Data Folder"="Raw_Data Folder") -> ()  [unwired: 10 in]
        n41 = case shown="\"PulseBlaster\", Default" "What To Change" {
          tunnel: w110 -> [w125 w168]
          tunnel: [w123 w167] -> w109
          tunnel: w108 -> [w124 w163]
          tunnel: w107 -> [w122 w165]
          tunnel: [w121 w166] -> w106
          tunnel: w101 -> [_ w164]
          tunnel: w101 -> [w120 _]
          tunnel: w100 -> [w119 w161]
          tunnel: w99 -> [w118 w160]
          tunnel: [w117 w159] -> w98
          tunnel: [w116 w158] -> w97
          frame "PulseBlaster", Default {
            n42 = for {
              tunnel: w124 -> [w136] mode=indexing
              shift-right: [w147] -> w123
              shift-left: w125 -> [w153]
              shift-right: [w129] -> w121
              shift-left: w122 -> [w150]
              tunnel: w120 -> [w141]
              shift-right: [w128] -> w117
              shift-left: w119 -> [w133]
              shift-right: [w127] -> w116
              shift-left: w118 -> [w132]
              i -> [w144]
              n43 = Unbundle By Name(w153) -> ("Instructions"=w155:T2)
              n44 = Multiply(x=1000.0, y=w136) -> (x*y=w134:dbl)
              n45 = Index Array(array=w155, index="PB Instruction Time To Change") -> (element=w157:T15)
              n46 = Bundle By Name(cluster=w157, "Time (s)"=w136) -> (w156:T15)
              n47 = Replace Array Subset(array=w155, new element=w156, index="PB Instruction Time To Change") -> (w152:T2)
              n48 = local read "Acquisition Parameters"() -> (w146:T4)
              n49 = Bundle By Name(cluster=w153, "Instructions"=w152) -> (w151:T13)
              n50 = local read "Camera Information"() -> (w145:T3)
              n51 = local read "Raw_Data Folder"() -> (w139:path)
              n52 = call "WriteExp.vi"("error in (no error)"=w150, "Control Task In"=w133, "Waveform Task In"=w132, "Experimental Control Cluster In"=w151) -> ("error out"=w149:errorcluster, "waveform task out"=w127:refnum<k21>, "counter task out"=w131:refnum<k21>, "Experimental Control Cluster Out"=w148:T13)  [unwired: 4 in]
              n53 = call "DoExperiment.vi"("Error In"=w149, "Camera Information 2"=w145, "Acquisition Parameters"=w146, "output cluster"=w148) -> ("error out"=w130:errorcluster, "Background Image"=w143:i32[][], "Atom Image"=w142:i32[][], "output cluster 2"=w147:T13)  [unwired: 4 in]
              n54 = Increment(x=w144) -> (x+1=w140:i32)
              n55 = call <vilib>:"DAQmx Wait Until Done.vi"("task/channels in"=w131, "error in"=w130) -> ("task out"=w128:refnum<k21>, "error out"=w129:errorcluster)  [unwired: 12 in]
              n56 = call "SaveImages.vi"("Background Image"=w143, "Atoms Image"=w142, "Base Filename"=w141, "Raw Data Path"=w139, "ImageNumber"=w140) -> ("Background Image 2"=→"Background Image":i16[][], "Atoms Image 2"=→"Atom Image":i16[][])  [unwired: 9 in]
              n57 = call "WriteBatches.vi"("Variable Parameter Value"=w134, "Image Number"=w140, "String"=w141, "Raw Data Folder"=w139) -> ()  [unwired: 8 in]
            }
            n58 = local write "You Are Changing:"("A Pulseblaster Param" ("You Are Changing:")) -> ()
          }
          frame "Static Voltage" {
            n59 = Array Size(array=w163) -> (size(s)=w162:i32)
            n60 = for {
              shift-right: [w188] -> w167
              shift-left: w168 -> [w196]
              tunnel: w163 -> [w187] mode=indexing
              shift-right: [w170] -> w166
              shift-left: w165 -> [w190]
              tunnel: w164 -> [w181]
              tunnel: w162 -> [w179]
              shift-right: [w173] -> w159
              shift-left: w161 -> [w176]
              shift-right: [w172] -> w158
              shift-left: w160 -> [w175]
              i -> [w178]
              n61 = Unbundle By Name(w196) -> ("6704 Static Voltage Settings.Voltages"=w197:dbl[])
              n62 = Replace Array Subset(array=w197, new element=w187, index="Static Channel To Change") -> (w195:dbl[])
              n63 = Bundle By Name(cluster=w196, "6704 Static Voltage Settings.Voltages"=w195) -> (w194:T13)
              n64 = local read "Acquisition Parameters"() -> (w192:T4)
              n65 = local read "Camera Information"() -> (w191:T3)
              n66 = local read "Raw_Data Folder"() -> (w186:path)
              n67 = call "WriteExp.vi"("error in (no error)"=w190, "Control Task In"=w176, "Waveform Task In"=w175, "Experimental Control Cluster In"=w194) -> ("error out"=w189:errorcluster, "waveform task out"=w172:refnum<k21>, "counter task out"=w174:refnum<k21>, "Experimental Control Cluster Out"=w193:T13)  [unwired: 4 in]
              n68 = call "DoExperiment.vi"("Error In"=w189, "Camera Information 2"=w191, "Acquisition Parameters"=w192, "output cluster"=w193) -> ("error out"=w171:errorcluster, "Background Image"=w185:i32[][], "Atom Image"=w184:i32[][], "output cluster 2"=w188:T13)  [unwired: 4 in]
              n69 = Increment(x=w178) -> (x+1=w177:i32)
              n70 = call "WriteBatches.vi"("Variable Parameter Value"=w187, "Image Number"=w177, "String"=w181, "Raw Data Folder"=w186) -> ()  [unwired: 8 in]
              n71 = call "Progress Bar.vi"("Total Number"=w179, "Current Number"=w177) -> ("Scan Progress"=→"Scan Progress":dbl)  [unwired: 13 in]
              n72 = call "SaveImages.vi"("Background Image"=w185, "Atoms Image"=w184, "Base Filename"=w181, "Raw Data Path"=w186, "ImageNumber"=w177) -> ("Background Image 2"=w183:i16[][], "Atoms Image 2"=w182:i16[][])  [unwired: 9 in]
              n73 = call <vilib>:"DAQmx Wait Until Done.vi"("task/channels in"=w174, "error in"=w171) -> ("task out"=w173:refnum<k21>, "error out"=w170:errorcluster)  [unwired: 12 in]
              n74 = local write "Background Image"(w183) -> ()
              n75 = local write "Atom Image"(w182) -> ()
            }
            "You Are Changing:" <- "A Static Voltage" ("You Are Changing:")
          }
        }
        "error constant" <- w106
        n76 = local write "Start Experiment"(FALSE ("Start Experiment")) -> ()
      }
      frame "Load Experiment" {
      }
      frame "Shutdown" {
        n77 = call <userlib>:"ShutDown.vi"("error in (no error)"=w206) -> ("error out"=w202:errorcluster)  [unwired: 1 in, 1 out]
        n78 = property on="Camera Ready" class="Bool (strict)"(error in=w202, "Value"=FALSE ("Camera Ready")) -> (error out=w201:errorcluster)  [unwired: 1 in, 1 out]
        n79 = local write "Shutdown Experiment"(FALSE ("Shutdown Experiment")) -> ()
      }
    }
  }
